vi "Make_Preference_b-n_101_with_without_Elong-1.vi"(4 "error IN":errorcluster, 7 "[IN] Subtracks in Row":T1(array[cluster])) -> (0 "error OUT":errorcluster, 3 "[OUT Subtracks in Row":T1(array[cluster]))   [LabVIEW 2013]
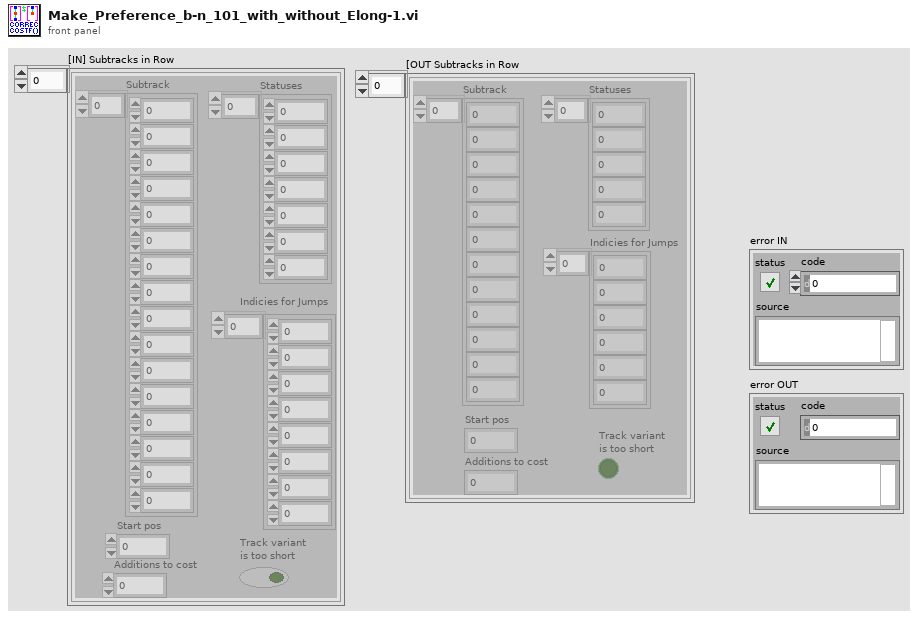
[diagram p1: front panel]
types:
  T1 = cluster{"Subtrack":dbl[], "Statuses":i16[], "Start pos":i32, "Additions to cost":i8, "Track variant \nis too short":bool, "Indicies for Jumps":i32[]}[]
  T2 = cluster{"Subtrack":dbl[], "Statuses":i16[], "Start pos":i32, "Additions to cost":i8, "Track variant \nis too short":bool, "Indicies for Jumps":i32[]}
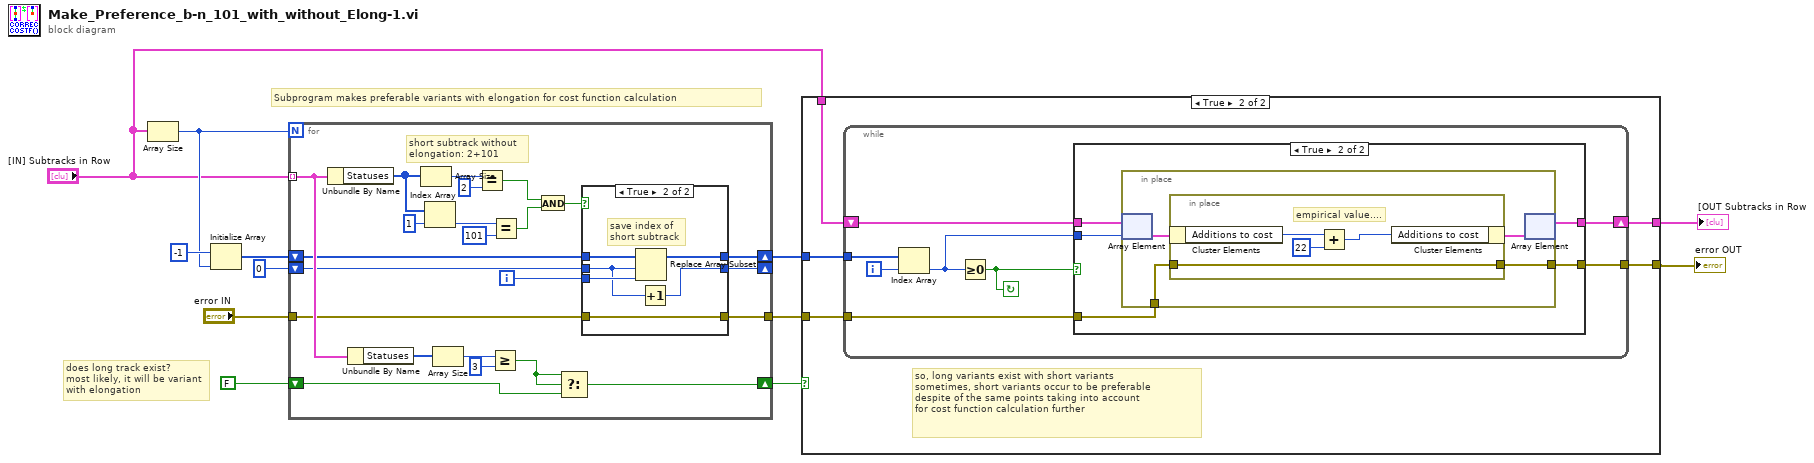
[diagram p0: block diagram]
diagram:
  # "Subprogram makes preferable variants with elongation for cost function calculation"
  # "does long track exist? \nmost likely, it will be variant\nwith elongation"
  n1 = Array Size(array="[IN] Subtracks in Row") -> (size(s)=w10:i32)
  n2 = Initialize Array(-1 ("element"), w10) -> (w9:i32[])
  n3 = for {
    N: w10 -> [_]
    tunnel: "[IN] Subtracks in Row" -> [w27] mode=indexing
    shift-right: [w14] -> w6
    shift-left: FALSE -> [w13]
    shift-right: [w18] -> w3
    shift-left: w9 -> [w22]
    shift-right: [w19] -> _
    shift-left: 0 -> [w21]
    tunnel: "error IN" -> [w17]
    tunnel: [w16] -> w4
    i -> [w20]
    # "short subtrack without\nelongation: 2+101"
    n4 = Unbundle By Name(w27) -> ("Statuses"=w33:i16[])
    n5 = Unbundle By Name(w27) -> ("Statuses"=w26:i16[])
    n6 = Array Size(array=w33) -> (size(s)=w35:i32)
    n7 = Index Array(array=w33, index=1) -> (element=w31:i16)
    n8 = Array Size(array=w26) -> (size(s)=w25:i32)
    n9 = Equal?(x=w35, y=2) -> (x = y?=w29:bool)
    n10 = Greater Or Equal?(x=w25, y=3) -> (x >= y?=w15:bool)
    n11 = Equal?(x=w31, y=i16 101) -> (x = y?=w28:bool)
    n12 = And(x=w29, y=w28) -> (x .and. y?=w23:bool)
    n13 = Select(t=w15, s=w15, f=w13) -> (s? t:f=w14:bool)
    n14 = case shown="True" w23 {
      tunnel: w22 -> [w38 w44]
      tunnel: w21 -> [w37 w42]
      tunnel: w20 -> [_ w43]
      tunnel: [w37 w41] -> w19
      tunnel: [w38 w40] -> w18
      tunnel: w17 -> [w36 w39]
      tunnel: [w36 w39] -> w16
      frame False {
      }
      frame True {
        # "save index of \nshort subtrack"
        n15 = Replace Array Subset(array=w44, new element=w43, index=w42) -> (w40:i32[])
        n16 = Increment(x=w42) -> (x+1=w41:i32)
      }
    }
  }
  n17 = case shown="True" w6 {
    tunnel: "[IN] Subtracks in Row" -> [w45 w49]
    tunnel: w4 -> [w46 w51]
    tunnel: w3 -> [_ w50]
    tunnel: [w46 w48] -> w2
    tunnel: [w45 w47] -> w1
    frame False {
      # "all tracks are: or long enough,\neither all of them are short"
    }
    frame True {
      # "so, long variants exist with short variants\nsometimes, short variants occur to be preferable\ndespite of the same points taking into account \nfor cost function calculation further"
      n18 = while {
        tunnel: w51 -> [w53]
        tunnel: w50 -> [w59]
        shift-right: [w54] -> w47
        shift-left: w49 -> [w57]
        tunnel: [w52] -> w48
        i -> [w58]
        stop <- w55 continue-if-true
        n19 = Index Array(array=w59, index=w58) -> (element=w56:i32)
        n20 = Greater Or Equal To 0?(x=w56) -> (x >= 0?=w55:bool)
        n21 = case shown="True" w55 {
          tunnel: w57 -> [w61 w66]
          tunnel: w56 -> [_ w65]
          tunnel: [w61 w63] -> w54
          tunnel: w53 -> [w60 w64]
          tunnel: [w60 w62] -> w52
          frame False {
          }
          frame True {
            n22 = in-place {
              in-place-border: w64 -> [w69]
              in-place-border: [w67] -> w62
              n23 = in-place-array #1(w66, w65) -> (w70:T2)
              n24 = in-place {
                in-place-border: w69 -> [w71]
                in-place-border: [w71] -> w67
                # "empirical value...."
                n25 = in-place-cluster #2(w70) -> ("Additions to cost"=w74:i8)
                n26 = Add(x=w74, y=i8 22) -> (x+y=w73:i8)
                n27 = in-place-cluster #2("Additions to cost"=w73) -> (w68:T2)
              }
              n28 = in-place-array #1(w68) -> (w63:T1)  [unwired: 1 out]
            }
          }
        }
      }
    }
  }
  "error OUT" <- w2
  "[OUT Subtracks in Row" <- w1
